vi "Autonomous.vi"   [LabVIEW 2018]
doc: "This VI starts when autonomous period begins, and will automatically be terminated when it ends. You can carry out timed or sensor driven operations directly to I/O or to subsystems without needing to return to the caller."
uses:
  Drive/Implementation/Drive Operations.ctl
  Support Code/Path Data.ctl
  Framework/Robot Global Data.vi
  <vilib>/Rock Robotics/Network Tables/NT Read String.vi
types:
  T1 = typedef "Path Data.ctl" = cluster{"Maneuver":enum16{"MAX 90", "MAX 180", "Turn to Home", "Turn to Rocket", "Auto-Align", "Turn to ..."}, "Rotation Direction":enum16{"N/A", "Right", "Left"}}[]
  T2 = typedef "Drive Operations.ctl" = enum16{"Reserve", "Read Current", "Immediate", "J-Turn", "Play Back From Log", "Auto-Align"}
  T3 = typedef "WPI_JoystickDevRef.ctl" = cluster{"Device":T4}
  T4 = typedef "WPI_JoystickDeviceEnum.ctl" = enum16{"USB 0", "USB 1", "USB 2", "USB 3", "USB 4", "USB 5"}
  T5 = typedef "Command Status Info.ctl" = cluster{"Name":string, "Status":T6, "notifier out":T7}
  T6 = typedef "Completion Status.ctl" = enum16{"Successful", "Aborted", "Incomplete"}
  T7 = typedef "Completion Notifier.ctl" = refnum<notifier>
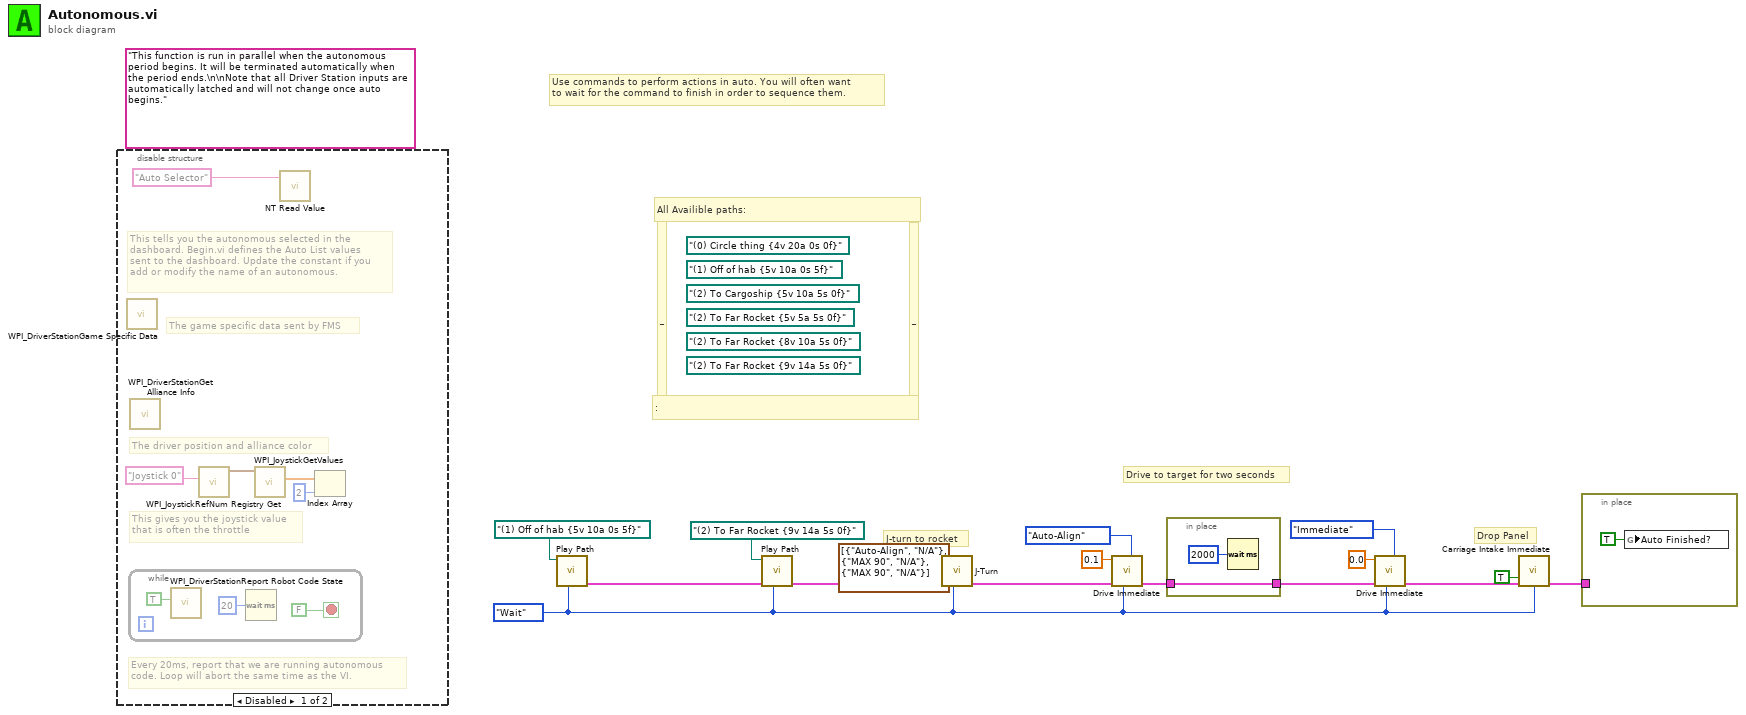
[diagram p0: block diagram]
diagram:
  (unwired) path "(2) To Far Rocket {5v 5a 5s 0f}"
  (unwired) path "(2) To Far Rocket {8v 10a 5s 0f}"
  (unwired) path "(2) To Cargoship {5v 10a 5s 0f}"
  (unwired) path "(2) To Far Rocket {9v 14a 5s 0f}"
  (unwired) path "(1) Off of hab {5v 10a 0s 5f}"
  w6 = enum16{"Start", "Wait"}."Wait" ("Synchronication")
  (unwired) path "(0) Circle thing {4v 20a 0s 0f}"
  (unwired) "This function is run in parallel when the autonomous period begins. It will be terminated automatically when the period ends.\n\nNote that all Driver Station inputs are automatically latched and will not change once auto begins."
  # "Drop Panel"
  # "Drive to target for two seconds"
  # ":"
  # "_"
  # "_"
  # "All Availible paths:"
  # "J-turn to rocket"
  # "Use commands to perform actions in auto. You will often want\nto wait for the command to finish in order to sequence them."
  n1 = disable-structure shown="Disabled" {
    frame Disabled {
      # "The game specific data sent by FMS"
      # "This tells you the autonomous selected in the \ndashboard. Begin.vi defines the Auto List values\nsent to the dashboard. Update the constant if you\nadd or modify the name of an autonomous."
      # "Every 20ms, report that we are running autonomous\ncode. Loop will abort the same time as the VI."
      # "This gives you the joystick value\nthat is often the throttle"
      # "The driver position and alliance color"
      n2 = call <vilib>:"WPI_DriverStationGame Specific Data.vi"() -> ()  [unwired: 11 in, 1 out]
      n3 = while {
        stop <- FALSE stop-if-true
        n4 = call <vilib>:"WPI_DriverStationReport Robot Code State.vi"("Autonomous"=TRUE) -> ()  [unwired: 10 in, 1 out]
        n5 = Wait (ms)(milliseconds to wait=u32 20) -> ()  [unwired: 1 out]
      }
      n6 = call <vilib>:"WPI_DriverStationGet Alliance Info.vi"() -> ()  [unwired: 12 out]
      n7 = call <vilib>:"WPI_JoystickRefNum Registry Get.vi"("refnum name"="Joystick 0") -> ("JoystickDevRef"=w20:T3)  [unwired: 1 in, 9 out]
      n8 = call <vilib>:"WPI_JoystickGetValues.vi"("JoystickDevRef"=w20) -> ("Axes"=w19:dbl[])  [unwired: 6 in, 4 out]
      n9 = call-poly <vilib>:"NT Read Value.vi"("Name"="Auto Selector") -> ()  [unwired: 9 in, 2 out]
      n10 = Index Array(array=w19, index=2) -> ()  [unwired: 1 out]
    }
    frame Enabled {
    }
  }
  n11 = call "Play Path.vi"("Synchronication"=w6, "Path"=path "(1) Off of hab {5v 10a 0s 5f}") -> ("Command Info Out"=w14:T5)  [unwired: 9 in]
  n12 = call "Play Path.vi"("Synchronication"=w6, "Command Info In"=w14, "Path"=path "(2) To Far Rocket {9v 14a 5s 0f}") -> ("Command Info Out"=w1:T5)  [unwired: 8 in]
  n13 = call "J-Turn.vi"("Synchronication"=w6, "Command Info In"=w1, "Path Data"=T1 [{"Maneuver"=enum."Auto-Align", "Rotation Direction"=enum."N/A"}, {"Maneuver"=enum."MAX 90", "Rotation Direction"=enum."N/A"}, {"Maneuver"=enum."MAX 90", "Rotation Direction"=enum."N/A"}]) -> ("Command Info Out"=w12:T5)  [unwired: 8 in]
  n14 = call "Drive Immediate.vi"("Operation"=Drive_Operations."Auto-Align", "Synchronication"=w6, "Command Info In"=w12, "Left Setpoint (Power)"=0.1) -> ("Command Info Out"=w9:T5)  [unwired: 7 in]
  n15 = in-place {
    in-place-border: w9 -> [w26]
    in-place-border: [w26] -> w8
    n16 = Wait (ms)(milliseconds to wait=u32 2000) -> ()  [unwired: 1 out]
  }
  n17 = call "Drive Immediate.vi"("Operation"=Drive_Operations."Immediate", "Synchronication"=w6, "Command Info In"=w8, "Left Setpoint (Power)"=0.0) -> ("Command Info Out"=w7:T5)  [unwired: 7 in]
  n18 = call "Carriage Intake Immediate.vi"("Close"=TRUE, "Command Info In"=w7, "Synchronication"=w6) -> ("Command Info Out"=w16:T5)  [unwired: 12 in]
  n19 = in-place {
    in-place-border: w16 -> [_]
    n20 = global write "Robot Global Data.vi" "Auto Finished?"(TRUE ("Auto Finished?")) -> ()
  }
